vi "clearpath_check_send.vi"(2 "Message Type":i32, 3 "Ack List In":i32[](array[numeric]), 4 "New Data":bool) -> (0 "Ack List Out":i32[](array[numeric]), 1 "Add to Queue":bool)   [LabVIEW 2011, in "clearpath_interface.lvlib"]
doc: "Compares a message type with the list of unacknowledged transmissions and a new data indicator to see if a new message of the provided type needs to issued. If so, the message type will be inserted into the Ack List."
uses:
  clearpath_interface.lvlib
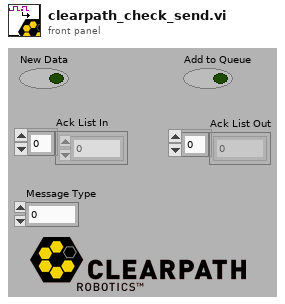
[diagram p1: front panel]
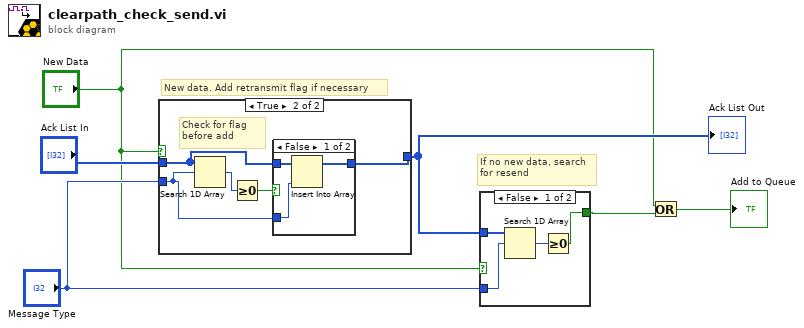
[diagram p0: block diagram]
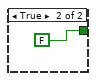
[diagram p2: hidden frame]
diagram:
  # "New data. Add retransmit flag if necessary"
  # "If no new data, search\nfor resend"
  n1 = case shown="True" "New Data" {
    tunnel: "Ack List In" -> [w7 w11]
    tunnel: [w7 w12] -> w4
    tunnel: "Message Type" -> [_ w10]
    frame False {
    }
    frame True {
      # "Check for flag before add"
      n2 = Search 1D Array(1D array=w11, element=w10) -> (index of element=w9:i32)  [unwired: 1 in]
      n3 = Greater Or Equal To 0?(x=w9) -> (x >= 0?=w8:bool)
      n4 = case shown="False" w8 {
        tunnel: w11 -> [w15 w16]
        tunnel: [w14 w16] -> w12
        tunnel: w10 -> [w13 _]
        frame False {
          n5 = Insert Into Array(array=w15, new element=w13) -> (w14:i32[])  [unwired: 1 in]
        }
        frame True {
        }
      }
    }
  }
  "Ack List Out" <- w4
  n6 = case shown="False" "New Data" {
    tunnel: "Message Type" -> [w20 _]
    tunnel: w4 -> [w18 _]
    tunnel: [w17 FALSE] -> w3
    frame False {
      n7 = Search 1D Array(1D array=w18, element=w20) -> (index of element=w19:i32)  [unwired: 1 in]
      n8 = Greater Or Equal To 0?(x=w19) -> (x >= 0?=w17:bool)
    }
    frame True {
    }
  }
  n9 = Or(x="New Data", y=w3) -> (x .or. y?=→"Add to Queue":bool)
